vi "mmf frame rate.vi"() -> ()   [LabVIEW 2010]
panel:
  in  "MMF Frame Rate":dbl
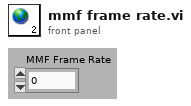
[diagram p1: front panel]
diagram:
